vi "PicoScope6000GetTimebase2.vi"(4 "Number of Samples":u32, 6 "Memory Segment":u32, 7 "Acquisition Settings":T1, 10 "handle in":i16, 11 "error in (no error)":errorcluster) -> (2 "handle out":i16, 3 "error out":errorcluster, 5 "Properties Panel":T3 {"Max Total Capture Time Available (sec)" format="%.3p"; "Sample Frequency" format="%.3p"; "Sample Internal" format="%.3p"; "Max Samples Available" format="%.3p"; "Total Capture Time (sec)" format="%.3p"})   [LabVIEW 2009]
uses:
  ps6000.dll
panel:
  in  "Acquisition SettingsBU":T2 {"Down Sample Ratio" min=1 step=1; "Down-Sample Mode" items=["None", "Aggregate", "Average", "Decimate", "Distribution"]}
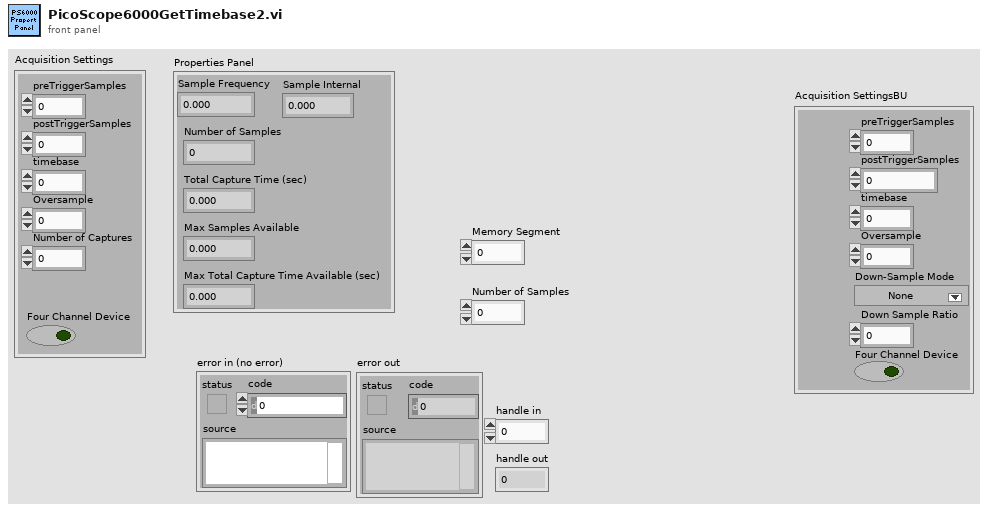
[diagram p1: front panel]
types:
  T1 = cluster{"preTriggerSamples":u32, "postTriggerSamples":u32, "timebase":u32, "Four Channel Device":bool, "Oversample":i16, "Number of Captures":u32}
  T2 = cluster{"preTriggerSamples":u32, "postTriggerSamples":u32, "timebase":u32, "Down-Sample Mode":i32, "Down Sample Ratio":u32, "Four Channel Device":bool, "Oversample":i16}
  T3 = cluster{"Sample Frequency":sgl, "Sample Internal":sgl, "maxSamples":u32, "Number of Samples":u32, "Total Capture Time (sec) ":sgl, "Max Total Capture Time Available (sec)":sgl}
  T4 = cluster{sgl, sgl, "maxSamples":i32, "Number of Samples":u32, sgl, sgl}
  T5 = cluster{sgl, sgl, "maxSamples":u32, "Number of Samples":u32, sgl, sgl}
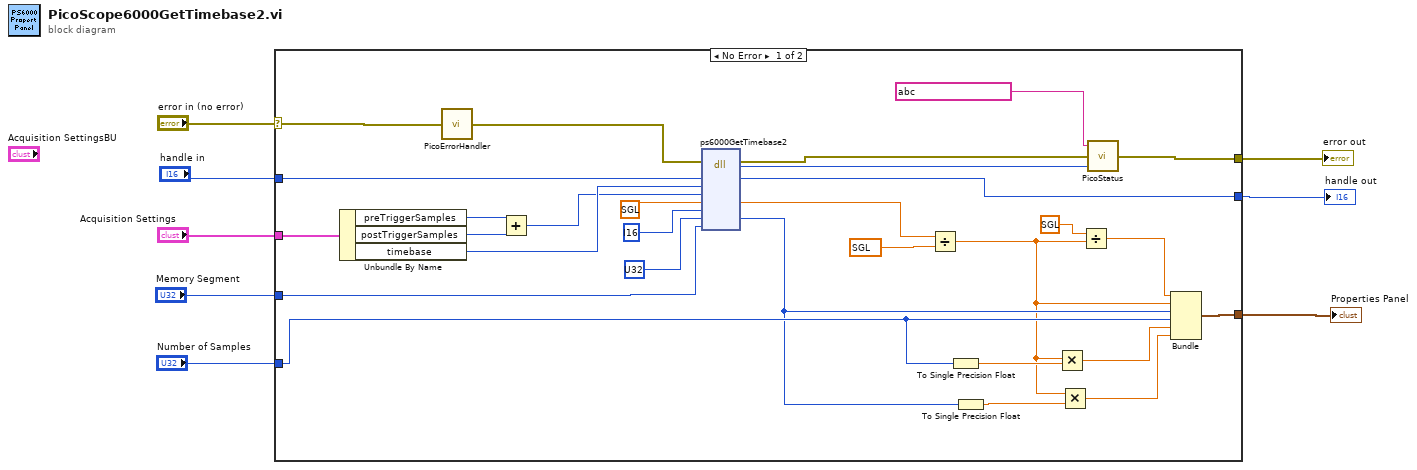
[diagram p0: block diagram]
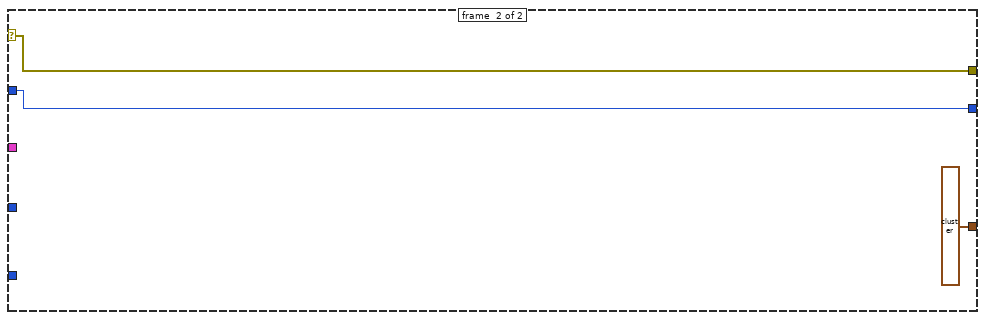
[diagram p2: hidden frame]
diagram:
  n1 = case shown="No Error" "error in (no error)" {
    selector: "error in (no error)" -> [w29 w40]
    tunnel: [w28 w40] -> w8
    tunnel: [w27 w39] -> w7
    tunnel: "Memory Segment" -> [w12 _]
    tunnel: "Number of Samples" -> [w22 _]
    tunnel: "handle in" -> [w26 w39]
    tunnel: "Acquisition Settings" -> [w25 _]
    tunnel: [w18 T4 ?] -> w2
    frame #0 {
      n2 = Unbundle By Name(w25) -> ("preTriggerSamples"=w31:u32, "postTriggerSamples"=w32:u32, "timebase"=w33:u32)
      n3 = call "PicoErrorHandler.vi"("error in"=w29) -> ("error out"=w35:errorcluster)
      n4 = Add(x=w31, y=w32) -> (x+y=w11:u32)
      n5 = dll-call lib="ps6000.dll" fn="ps6000GetTimebase2"(error in=w35, "handle"=w26, "timebase"=w33, "noSamples"=w11, "timeIntervalNanoseconds"=sgl ?, "oversample"=i16 ?, "maxSamples"=u32 ?, "segmentIndex"=w12) -> (error out=w34:errorcluster, "PICO_STATUS"=w30:u32, "handle"=w27:i16, "timeIntervalNanoseconds"=w36:sgl, "maxSamples"=w20:u32)  [unwired: 6 in, 1 out]
      n6 = Divide(x=w36, y=sgl ?) -> (x/y=w14:sgl)
      n7 = To Single Precision Float(number=w22) -> (single precision float=w24:sgl)
      n8 = To Single Precision Float(number=w20) -> (single precision float=w21:sgl)
      n9 = Multiply(x=w14, y=w24) -> (x*y=w23:sgl)
      n10 = Multiply(x=w14, y=w21) -> (x*y=w19:sgl)
      n11 = Divide(x=sgl ?, y=w14) -> (x/y=w15:sgl)
      n12 = call "PicoStatus.vi"("PICO STATUS"=w30, "error in"=w34, "source"=string ?) -> ("error out"=w28:errorcluster)
      n13 = Bundle(w15, w14, "maxSamples"=w20, "Number of Samples"=w22, w23, w19) -> (w18:T5)  [unwired: 1 in]
    }
    frame #1 {
    }
  }
  "error out" <- w8
  "handle out" <- w7
  "Properties Panel" <- w2
